vi "Read Registers to write.vi"(11 "Device in":refnum<class "PIC-Device.lvclass">) -> (2 "Registers to write":T1[](array[typedef]), 3 "Device out":refnum<class "PIC-Device.lvclass">)   [LabVIEW 2020, in "PIC-Device.lvclass"]
uses:
  PIC-Device.lvclass
  Controls/Register to Write.ctl
  PIC-Device.lvclass/PIC-Device.ctl
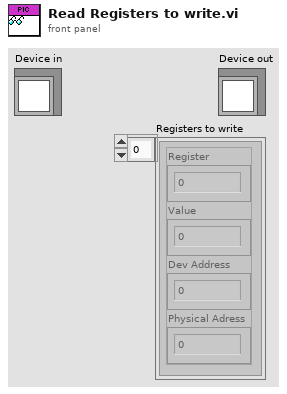
[diagram p1: front panel]
types:
  T1 = typedef "PIC-Device.lvclass/Register to Write.ctl" = cluster{"Register":u32, "Value":u32, "Dev Address":u32, "Physical Adress":u32}
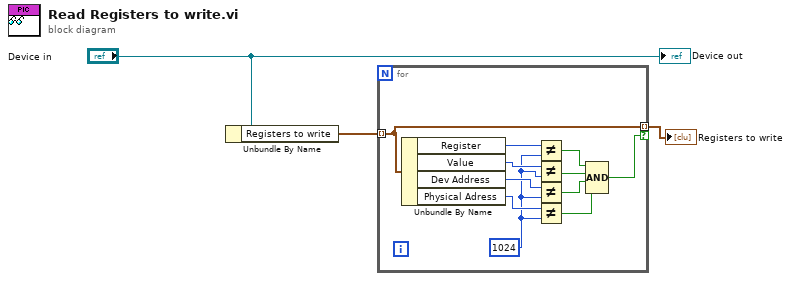
[diagram p0: block diagram]
diagram:
  n1 = Unbundle By Name("Device in") -> ("Registers to write"=w2:T1[])
  n2 = for {
    tunnel: w2 -> [w5] mode=indexing
    tunnel: [w5] -> w1 mode=indexing if=w4
    w10 = u32 1024
    n3 = Unbundle By Name(w5) -> ("Register"=w14:u32, "Value"=w13:u32, "Dev Address"=w12:u32, "Physical Adress"=w11:u32)
    n4 = Not Equal?(x=w14, y=w10) -> (x != y?=w9:bool)
    n5 = Not Equal?(x=w13, y=w10) -> (x != y?=w8:bool)
    n6 = Not Equal?(x=w12, y=w10) -> (x != y?=w7:bool)
    n7 = Not Equal?(x=w11, y=w10) -> (x != y?=w6:bool)
    n8 = Compound Arithmetic op=AND(w9, w8, w7, w6) -> (w4:bool)
  }
  "Registers to write" <- w1
  "Device out" <- "Device in"
